vi "Photon Counter barebones etch-a-sketch.vi"() -> ()   [LabVIEW 2023, in "Photon Counter.lvclass"]
uses:
  Photon Counter.lvclass
  SR400/SR400.lvlib
panel:
  in  "T_set (s)":dbl=0.3
  out "CPS":i32
  out "Minimum":i32
  out "Maximum":i32
  out "Counts":i32
  out "Waveform Chart":dbl(graph)
  in  "stop":bool
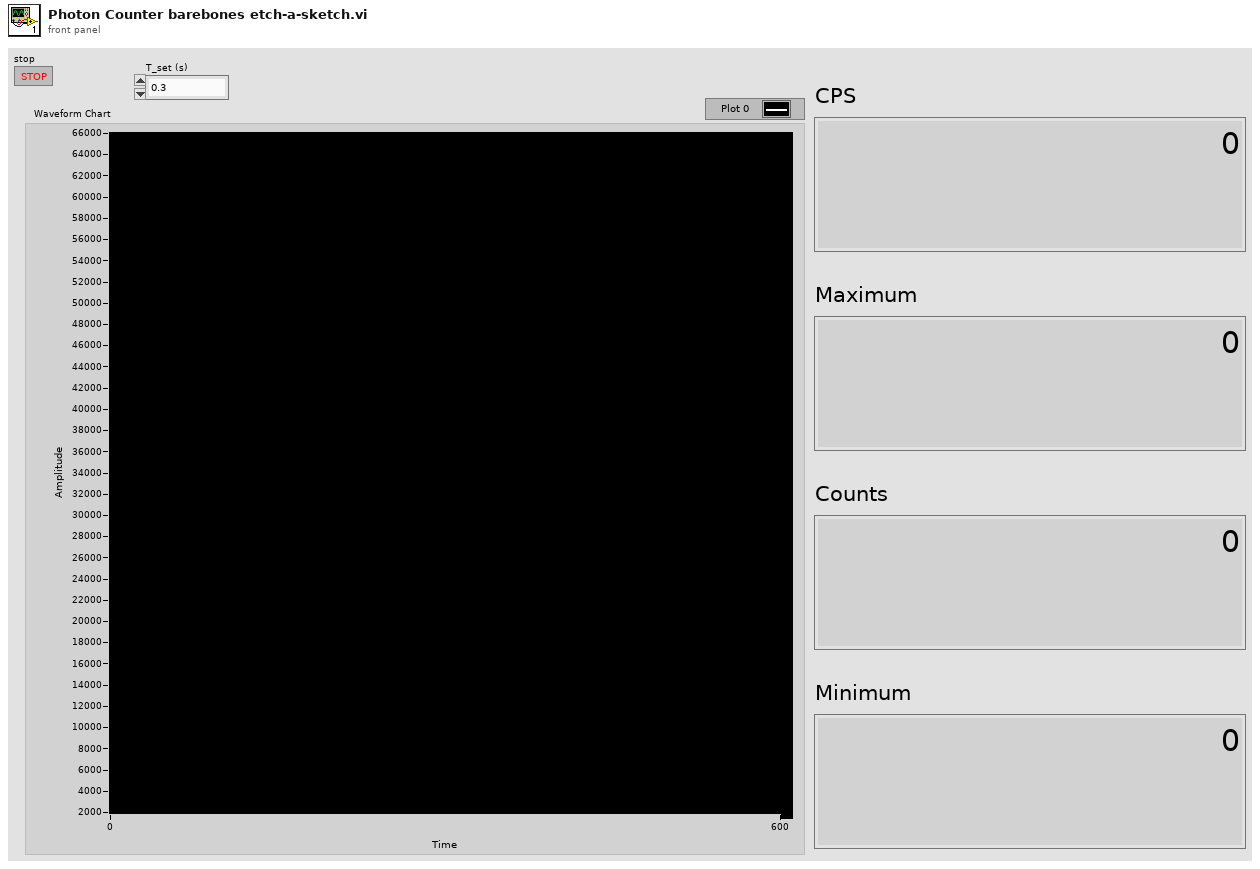
[diagram p1: front panel]
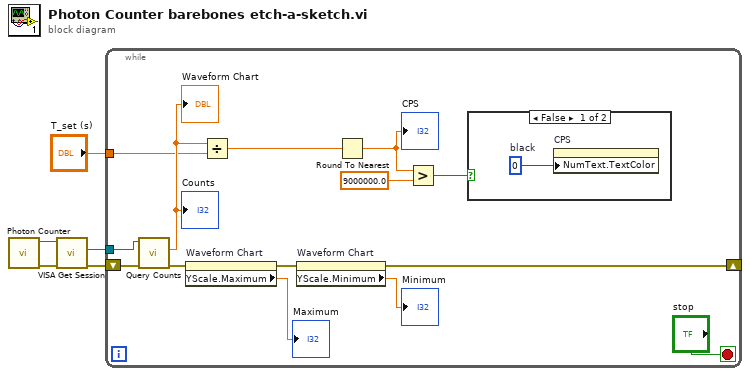
[diagram p0: block diagram]
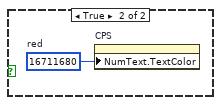
[diagram p2: hidden frame]
diagram:
  n1 = call "Photon Counter.vi"() -> ("error out"=w4:errorcluster, "Photon Counter SR400 out"=w5:refnum<class "Photon Counter.lvclass">)  [unwired: 10 in]
  n2 = call-dynamic "VISA Get Session.vi"("error in (no error)"=w4, "Instrument.lvclass in"=w5) -> ("error out"=w1:errorcluster, "VISA Resource Name"=w2:refnum<visa-resource-name>)  [unwired: 8 out]
  n3 = while {
    shift-right: [w15] -> _
    shift-left: w1 -> [w18]
    tunnel: w2 -> [w11]
    tunnel: "T_set (s)" -> [w10]
    stop <- "stop" stop-if-true
    n4 = call "Query Counts.vi"("error in (no error)"=w18, "VISA resource name"=w11) -> ("error out"=w16:errorcluster, "Counts"=w12:dbl)  [unwired: 1 in, 7 out]
    "Waveform Chart" <- w12
    "Counts" <- w12
    n5 = property on="Waveform Chart" class="WFChart (strict)"(error in=w16) -> (error out=w17:errorcluster, "YScale.Maximum"=→"Maximum":dbl)  [unwired: 1 in, 1 out]
    n6 = Divide(x=w12, y=w10) -> (x/y=w9:dbl)
    n7 = property on="Waveform Chart" class="WFChart (strict)"(error in=w17) -> (error out=w15:errorcluster, "YScale.Minimum"=→"Minimum":dbl)  [unwired: 1 in, 1 out]
    n8 = Round To Nearest(number=w9) -> (nearest integer value=w8:dbl)
    "CPS" <- w8
    n9 = Greater?(x=w8, y=9000000.0) -> (0:w6:bool)
    n10 = case shown="False" w6 {
      frame False {
        w20 = u32 0  # black
        n11 = property on="CPS" class="DigNum (strict)"("NumText.TextColor"=w20) -> ()  [unwired: 2 in, 2 out]
      }
      frame True {
        w21 = u32 16711680  # red
        n12 = property on="CPS" class="DigNum (strict)"("NumText.TextColor"=w21) -> ()  [unwired: 2 in, 2 out]
      }
    }
  }
